vi "Auto-Refresh Init.vi"(8 "error in (no error)":errorcluster, 11 "SimSyA in":refnum<class "SimSyA.lvclass">) -> (0 "error out":errorcluster, 3 "SimSyA out":refnum<class "SimSyA.lvclass">)   [LabVIEW 2014, in "SimSyA.lvlib" / "SimSyA.lvclass"]
uses:
  SimSyA.lvclass
  SimSyA.lvclass/SimSyA.ctl
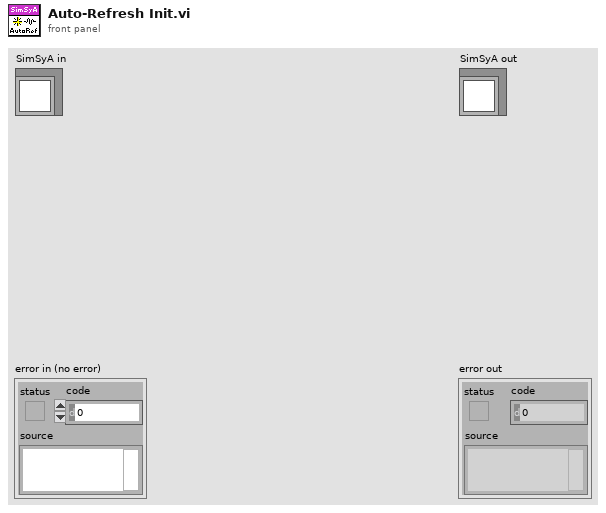
[diagram p1: front panel]
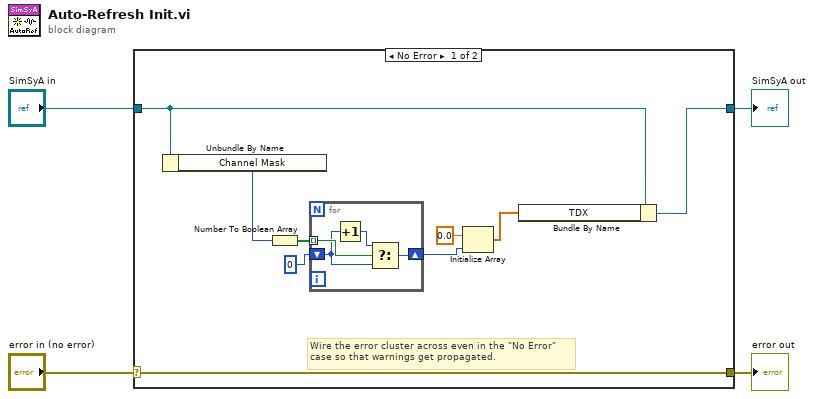
[diagram p0: block diagram]
diagram:
  n1 = case shown="No Error" "error in (no error)" {
    selector: "error in (no error)" -> [w13 w19]
    tunnel: [w13 w19] -> w3
    tunnel: [w12 w18] -> w1
    tunnel: "SimSyA in" -> [w6 w18]
    frame No Error {
      # "Wire the error cluster across even in the \"No Error\"\ncase so that warnings get propagated."
      n2 = Unbundle By Name(w6) -> ("Channel Mask"=w5:u64)
      n3 = Number To Boolean Array(number=w5) -> (Boolean array=w10:bool[])
      n4 = for {
        tunnel: w10 -> [w16] mode=indexing
        shift-right: [w17] -> w8
        shift-left: 0 -> [w14]
        n5 = Increment(x=w14) -> (x+1=w15:i32)
        n6 = Select(t=w15, s=w16, f=w14) -> (s? t:f=w17:i32)
      }
      n7 = Initialize Array(sgl 0.0 ("element"), w8) -> (w7:sgl[])
      n8 = Bundle By Name(cluster=w6, "TDX"=w7) -> (w12:refnum<class "SimSyA.lvclass">)
    }
    frame Error {
    }
  }
  "error out" <- w3
  "SimSyA out" <- w1
